vi "例13.3-2FFT.vi"() -> ()   [LabVIEW 2012]
uses:
  <vilib>/Analysis/4window.llb/windowTd.ctl
  <vilib>/Analysis/NI_AALPro.lvlib
panel:
  out "有效值":dbl
  in  "window":T1=1 caption="窗" items=["矩形"=0, "Hanning"=1, "Hamming"=2, "Blackman-Harris"=3, "Exact Blackman"=4, "Blackman"=5, "Flat Top"=6, "4阶Blackman-Harris "=7, "7阶Blackman-Harris"=8, "Low Sidelobe"=9, "Blackman Nuttall"=11, "三角"=30, "Bartlett-Hanning"=31, "Bohman"=32, "Parzen"=33, "Welch"=34, "Kaiser"=60, "Dolph-Chebyshev"=61, "高斯"=62]
  out "频率":dbl
  out "FFT":cluster{"f0":dbl, "df":dbl, "magnitude":dbl[]}(graph)
  in  "信噪比":dbl=1.0 format="%.2p"
  in  "相位":dbl
  in  "采样信息":cluster{"Fs":dbl, "#s":dbl}={"Fs"=1000.0, "#s"=1000.0}
  in  "幅值":dbl=1.0
  in  "频率":dbl=10.5
  in  "噪声选择":enum16{"无", "均匀白噪声", "高斯噪声"}(ring)
  out "波形图":waveform(dbl)(graph)
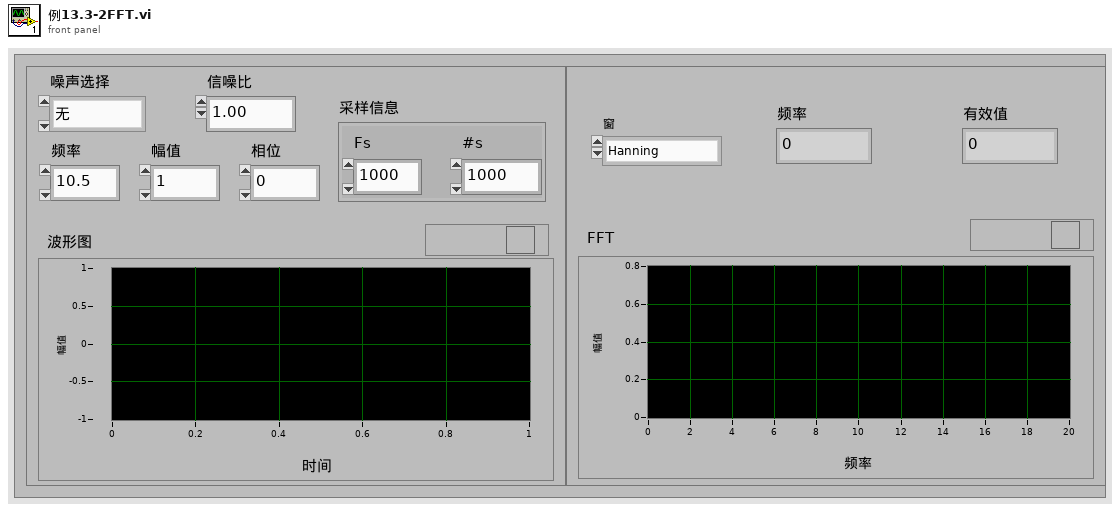
[diagram p1: front panel]
types:
  T1 = typedef "NI_AALPro.lvlib/windowTd.ctl" = u32
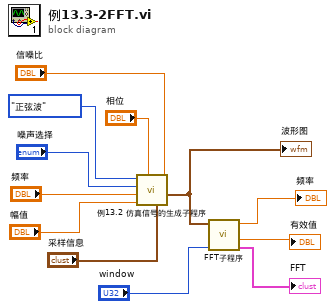
[diagram p0: block diagram]
diagram:
  n1 = call "例13.2 仿真信号的生成子程序.vi"("信噪比"="信噪比", "sampling info"="采样信息", "相位"="相位", "幅值"="幅值", "频率"="频率", "噪声选择"="噪声选择", "波形选择"=enum16{"正弦波", "三角波", "方波", "公式波"}."正弦波") -> ("波形图"=w1:waveform(dbl))  [unwired: 4 in]
  "波形图" <- w1
  n2 = call "FFT子程序.vi"("window"="window", "time signal"=w1) -> ("FFT幅值"=→"FFT":cluster{"f0":dbl, "df":dbl, "magnitude":dbl[]}, "频率的幅值"=→"有效值":dbl, "频率"=→"频率":dbl)  [unwired: 2 in, 1 out]
